vi "DSF.Engine.Plugin.Initialize Cache.vi"(8 "error in (no error)":errorcluster, 10 "Cache":refnum<class "DSF.Engine.Memory.Cache.lvclass">, 11 "Plugin in":refnum<class "DSF.Engine.Plugin.lvclass">) -> (0 "error out":errorcluster, 3 "Plugin out":refnum<class "DSF.Engine.Plugin.lvclass">)   [LabVIEW 2017]
uses:
  DSF.Engine.Plugin.lvclass
  Cache/DSF.Engine.Memory.Cache.lvclass
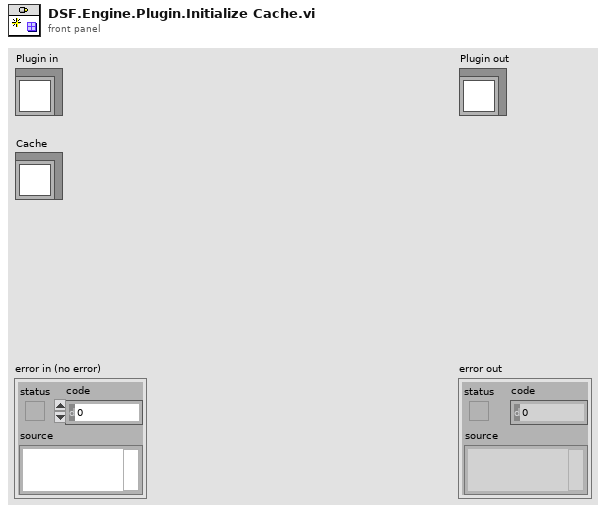
[diagram p1: front panel]
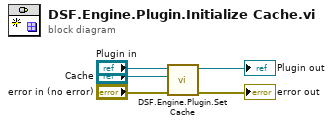
[diagram p0: block diagram]
diagram:
  n1 = call "DSF.Engine.Plugin.Set Cache.vi"("Cache"="Cache", "Plugin in"="Plugin in") -> ("Plugin out"=→"Plugin out":refnum<class "DSF.Engine.Plugin.lvclass">)  [unwired: 9 in]
  "error out" <- "error in (no error)"
